vi "Global - ADC.vi"() -> ()   [LabVIEW 2019]
panel:
  out "ADC":T1(array[cluster])
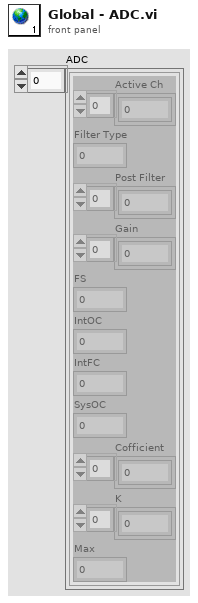
[diagram p1: front panel]
types:
  T1 = cluster{"Active Ch":u8[], "Filter Type":u8, "Post Filter":u8[], "Gain":u8[], "FS":u16, "IntOC":u8, "IntFC":u8, "SysOC":u8, "Cofficient":dbl[], "K":dbl[], "Max":i32}[]
diagram:
